vi "总计累积剂量计算-专用.vi"(11 "记录数组":string[][](array[string])) -> (3 "输出记录数组":string[][](array[string]))   [LabVIEW 2017]
panel:
  out "数值输入控件":dbl
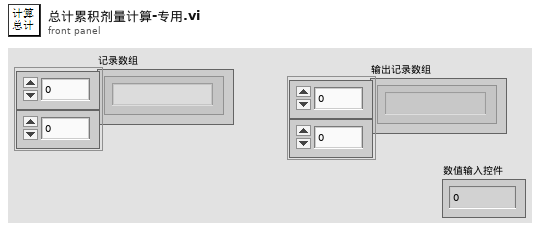
[diagram p1: front panel]
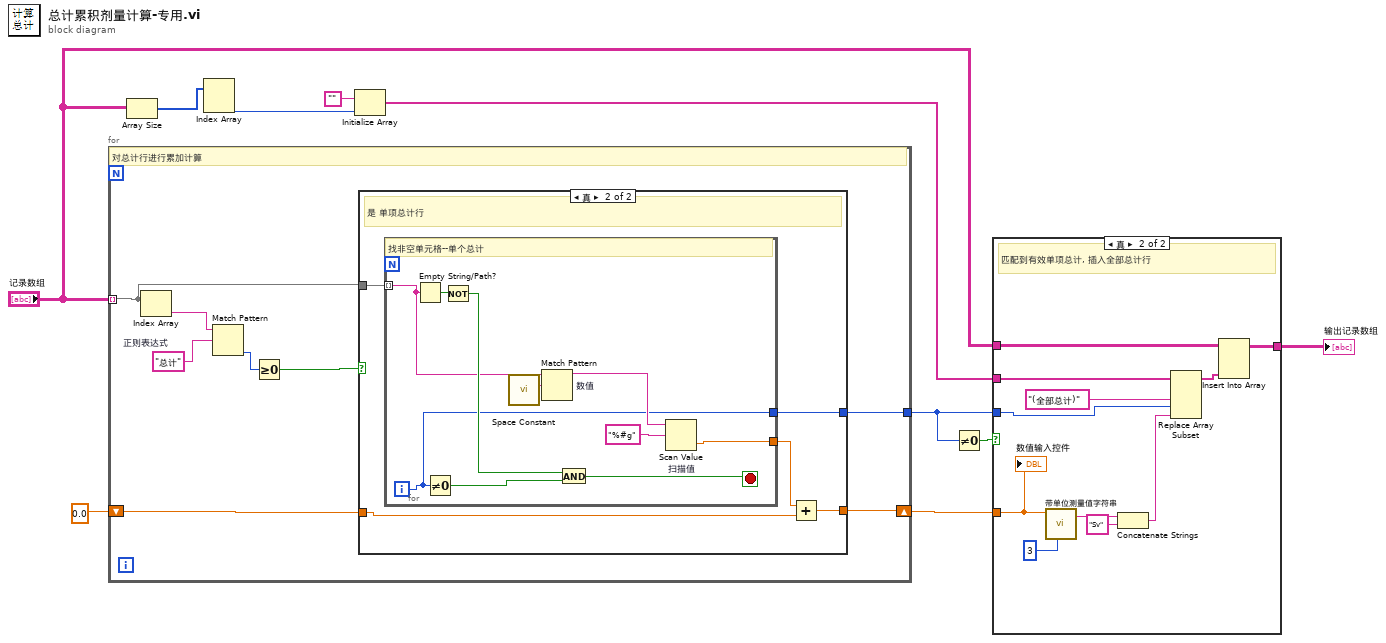
[diagram p0: block diagram]
diagram:
  n1 = for {
    tunnel: "记录数组" -> [w14] mode=indexing
    shift-right: [w12] -> w5
    shift-left: 0.0 -> [w13]
    tunnel: [w11] -> w2
    w17 = "总计"  # 正则表达式
    # "对总计行进行累加计算"
    n2 = Index Array(array=w14) -> (element=w18:string)  [unwired: 1 in]
    n3 = Match Pattern(string=w18, regular expression=w17) -> (offset past match=w16:i32)  [unwired: 1 in, 3 out]
    n4 = Greater Or Equal To 0?(x=w16) -> (x >= 0?=w15:bool)
    n5 = case shown="真" w15 {
      tunnel: w14 -> [_ w24]
      tunnel: w13 -> [w19 w22]
      tunnel: [w19 w21] -> w12
      tunnel: [_ w20] -> w11
      frame False {
      }
      frame True {
        # "是 单项总计行"
        n6 = for {
          tunnel: w24 -> [w30] mode=indexing
          tunnel: [w26] -> w23
          tunnel: [w25] -> w20
          i -> [w25]
          stop <- w31 stop-if-true
          # "找非空单元格--单个总计"
          n7 = Empty String/Path?(string/path=w30) -> (empty?=w34:bool)
          n8 = Not Equal To 0?(x=w25) -> (x != 0?=w33:bool)
          n9 = Not(x=w34) -> (.not. x?=w32:bool)
          n10 = call <vilib>:"Space Constant.vi"() -> ("String"=w29:string)
          n11 = Match Pattern "数值"(string=w30, regular expression=w29) -> (before substring=w28:string)  [unwired: 1 in, 3 out]
          n12 = And(x=w32, y=w33) -> (x .and. y?=w31:bool)
          n13 = Scan Value "扫描值"(string=w28, format string="%#g" ("格式字符串")) -> (value=w26:dbl)  [unwired: 1 in, 1 out]
        }
        n14 = Add(x=w23, y=w22) -> (x+y=w21:dbl)
      }
    }
  }
  n15 = Array Size(array="记录数组") -> (size(s)=w9:i32[])
  n16 = Index Array(array=w9) -> (element #2=w8:i32)  [unwired: 2 in, 1 out]
  n17 = Initialize Array("", w8) -> (w6:string[])
  n18 = Not Equal To 0?(x=w2) -> (x != 0?=w1:bool)
  n19 = case shown="真" w1 {
    tunnel: w6 -> [_ w46]
    tunnel: w5 -> [_ w44]
    tunnel: "记录数组" -> [w35 w39]
    tunnel: [w35 w37] -> w3
    tunnel: w2 -> [_ w36]
    frame False {
      # "未匹配到单项总计, 说明记录为空, 不计算总计"
    }
    frame True {
      # "匹配到有效单项总计, 插入全部总计行"
      n20 = call "带单位测量值字符串.vi"("精度(2)"=i16 3, "测量值"=w44) -> ("结果"=w42:string)  [unwired: 9 in]
      n21 = Concatenate Strings(w42, "Sv" ("字符串")) -> (w40:string)
      n22 = Replace Array Subset(array=w46, new element #1="(全部总计)", new element #2=w40, index #2=w36) -> (w38:string[])  [unwired: 1 in]
      n23 = Insert Into Array(array=w39, new element=w38) -> (w37:string[][])  [unwired: 2 in]
      "数值输入控件" <- w44
    }
  }
  "输出记录数组" <- w3
